vi "Programacion paralela.vi"() -> ()   [LabVIEW 2020]
panel:
  out "Thermometer 8":u8(slide) scale=0.0..100.0
  out "Thermometer 7":u8(slide) scale=0.0..100.0
  out "Thermometer 6":u8(slide) scale=0.0..100.0
  out "Thermometer 5":u8(slide) scale=0.0..100.0
  out "Thermometer 4":u8(slide) scale=0.0..100.0
  out "Thermometer 3":u8(slide) scale=0.0..100.0
  out "Thermometer 2":u8(slide) scale=0.0..100.0
  out "Thermometer":u8(slide) scale=0.0..100.0
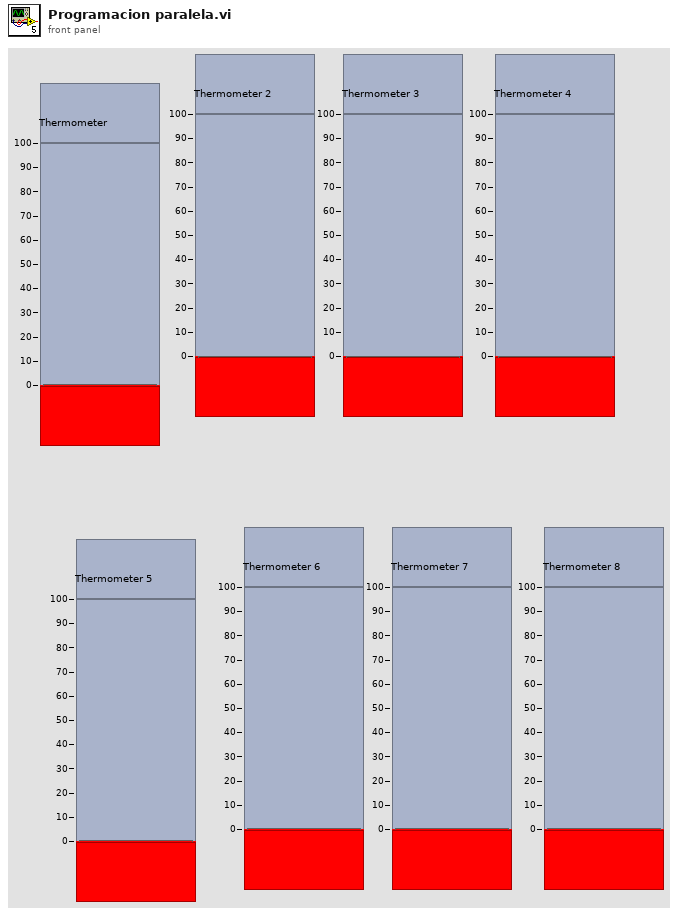
[diagram p1: front panel]
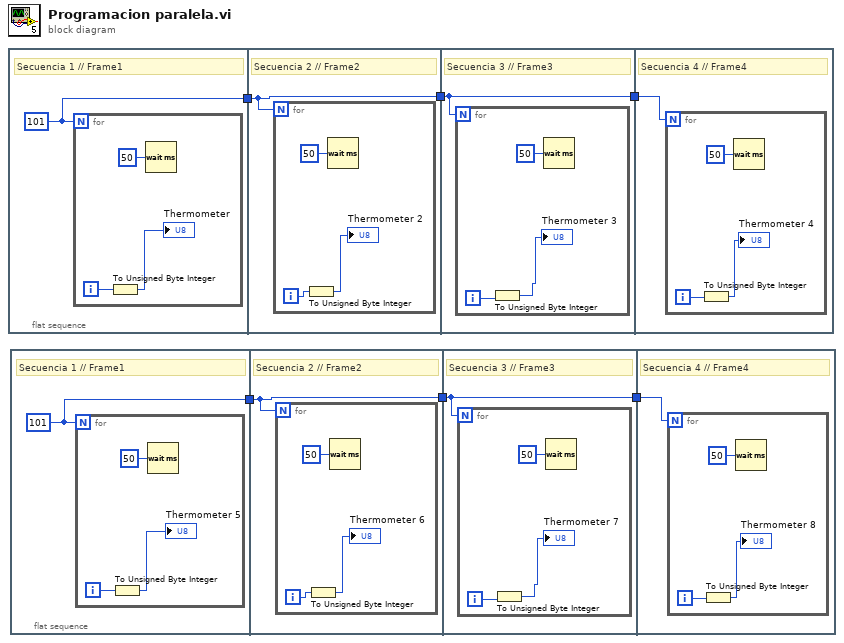
[diagram p0: block diagram]
diagram:
  n1 = flat-sequence {
    tunnel: [w7] -> w6
    tunnel: w6 -> [w11]
    tunnel: [w11] -> w5
    tunnel: w5 -> [w15]
    tunnel: [w15] -> w4
    tunnel: w4 -> [w19]
    frame #0 {
      w7 = 101
      # "Secuencia 1 // Frame1"
      n2 = for {
        N: w7 -> [_]
        i -> [w9]
        n3 = To Unsigned Byte Integer(number=w9) -> (unsigned 8bit integer=→"Thermometer":u8)
        n4 = Wait (ms)(milliseconds to wait=u32 50) -> ()  [unwired: 1 out]
      }
    }
    frame #1 {
      # "Secuencia 2 // Frame2"
      n5 = for {
        N: w11 -> [_]
        i -> [w14]
        n6 = To Unsigned Byte Integer(number=w14) -> (unsigned 8bit integer=→"Thermometer 2":u8)
        n7 = Wait (ms)(milliseconds to wait=u32 50) -> ()  [unwired: 1 out]
      }
    }
    frame #2 {
      # "Secuencia 3 // Frame3"
      n8 = for {
        N: w15 -> [_]
        i -> [w18]
        n9 = To Unsigned Byte Integer(number=w18) -> (unsigned 8bit integer=→"Thermometer 3":u8)
        n10 = Wait (ms)(milliseconds to wait=u32 50) -> ()  [unwired: 1 out]
      }
    }
    frame #3 {
      # "Secuencia 4 // Frame4"
      n11 = for {
        N: w19 -> [_]
        i -> [w22]
        n12 = To Unsigned Byte Integer(number=w22) -> (unsigned 8bit integer=→"Thermometer 4":u8)
        n13 = Wait (ms)(milliseconds to wait=u32 50) -> ()  [unwired: 1 out]
      }
    }
  }
  n14 = flat-sequence {
    tunnel: [w23] -> w3
    tunnel: w3 -> [w27]
    tunnel: [w27] -> w2
    tunnel: w2 -> [w31]
    tunnel: [w31] -> w1
    tunnel: w1 -> [w35]
    frame #0 {
      w23 = 101
      # "Secuencia 1 // Frame1"
      n15 = for {
        N: w23 -> [_]
        i -> [w25]
        n16 = To Unsigned Byte Integer(number=w25) -> (unsigned 8bit integer=→"Thermometer 5":u8)
        n17 = Wait (ms)(milliseconds to wait=u32 50) -> ()  [unwired: 1 out]
      }
    }
    frame #1 {
      # "Secuencia 2 // Frame2"
      n18 = for {
        N: w27 -> [_]
        i -> [w30]
        n19 = To Unsigned Byte Integer(number=w30) -> (unsigned 8bit integer=→"Thermometer 6":u8)
        n20 = Wait (ms)(milliseconds to wait=u32 50) -> ()  [unwired: 1 out]
      }
    }
    frame #2 {
      # "Secuencia 3 // Frame3"
      n21 = for {
        N: w31 -> [_]
        i -> [w34]
        n22 = To Unsigned Byte Integer(number=w34) -> (unsigned 8bit integer=→"Thermometer 7":u8)
        n23 = Wait (ms)(milliseconds to wait=u32 50) -> ()  [unwired: 1 out]
      }
    }
    frame #3 {
      # "Secuencia 4 // Frame4"
      n24 = for {
        N: w35 -> [_]
        i -> [w38]
        n25 = To Unsigned Byte Integer(number=w38) -> (unsigned 8bit integer=→"Thermometer 8":u8)
        n26 = Wait (ms)(milliseconds to wait=u32 50) -> ()  [unwired: 1 out]
      }
    }
  }
